vi "Test.vi"() -> ()   [LabVIEW 2020]
panel:
  out "error out":errorcluster
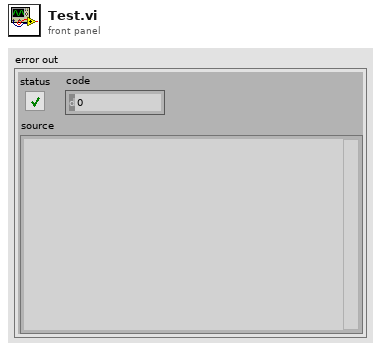
[diagram p1: front panel]
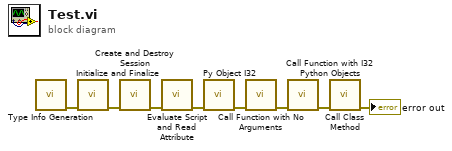
[diagram p0: block diagram]
diagram:
  n1 = call "Type Info Generation.vi"() -> ("error out"=w3:errorcluster)  [unwired: 11 in]
  n2 = call "Initialize and Finalize.vi"("error in (no error)"=w3) -> ("error out"=w8:errorcluster)  [unwired: 10 in]
  n3 = call "Create and Destroy Session.vi"("error in (no error)"=w8) -> ("error out"=w7:errorcluster)  [unwired: 10 in]
  n4 = call "Evaluate Script and Read Attribute.vi"("error in (no error)"=w7) -> ("error out"=w6:errorcluster)  [unwired: 10 in]
  n5 = call "Py Object I32.vi"("error in (no error)"=w6) -> ("error out"=w5:errorcluster)  [unwired: 10 in]
  n6 = call "Call Function with No Arguments.vi"("error in (no error)"=w5) -> ("error out"=w2:errorcluster)  [unwired: 10 in]
  n7 = call "Call Function with I32 Python Objects.vi"("error in (no error)"=w2) -> ("error out"=w4:errorcluster)  [unwired: 10 in]
  n8 = call "Call Class Method.vi"("error in (no error)"=w4) -> ("error out"=→"error out":errorcluster)  [unwired: 10 in]
